vi "termalImage 01.vi"() -> ()   [LabVIEW 2018]
doc: "This example performs writes and reads on a serial port, as directed by the user. You can press the Write and Read buttons, and change the Read Count, while the example is running.\n\nThe parameters set for the serial port must match the parameters of the connected instrument or device. In this example, the Read Count parameter specifies the number of bytes that the serial port reads. If there were more bytes at the port than the specified number, those bytes would not be read. If there were less bytes at the port than the specified number, you would receive a timeout error.\n\nThis example expands upon the flow control options for XON and XOFF, allowing the user to choose those control characters. Also, the user can enable or disable a termination character. Some devices require a termination character in order to identify the end of command strings. Some devices send a termination character to signify the end of data to be read. This example shows how you can end the Read operation once a termination character is detected in the buffer and/or append a termination character at the end of the Write data."
uses:
  <vilib>/userdefined/High Color/IMAQdx.ctl
  <vilib>/Instr/_visa.llb/VISA Configure Serial Port (Instr).vi
  <vilib>/vision/driver/NI_Vision_Acquisition_Software.lvlib
  <vilib>/vision/NI_Vision_Development_Module.lvlib
panel:
  out "Cam  2":T1(plugin-control)
  in  "Camera":T2="cam1"
  in  "stop":bool
  in  "stop 2":bool
  in  "폭":dbl=10.0
  in  "중심":dbl=35.0
  out "Temperature":dbl[][](graph)
  in  "Stop":bool
  in  "VISA resource name":refnum<visa-resource-name>="COM6"
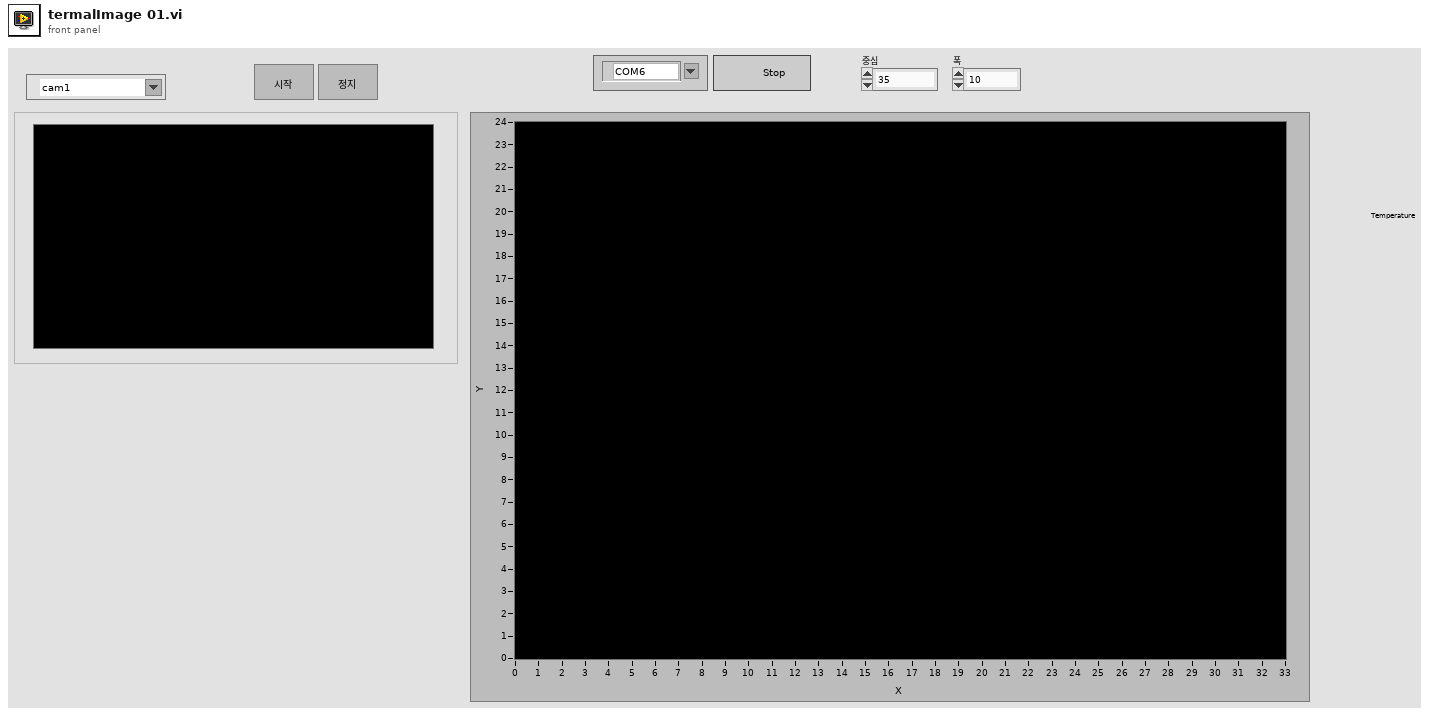
[diagram p1: front panel]
types:
  T1 = typedef "IMAQ Image.ctl" = refnum<image>
  T2 = typedef "IMAQdx.ctl" = refnum<k21>
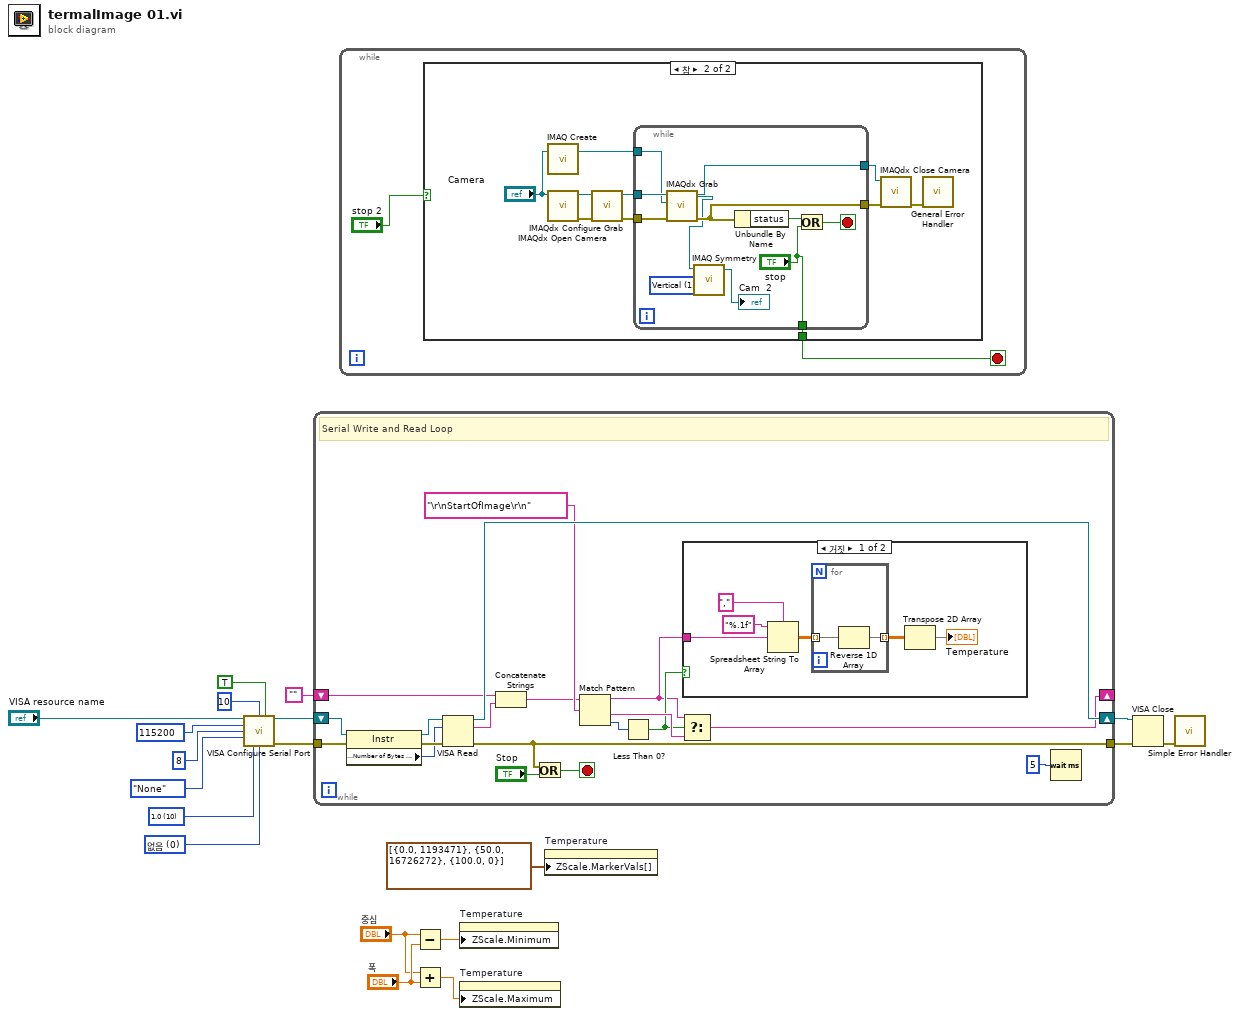
[diagram p0: block diagram]
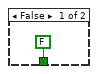
[diagram p2: hidden frame]
diagram:
  w6 = u16 0 items=["없음", "XON/XOFF", "RTS/CTS", "XON/XOFF & RTS/CTS", "DTR/DSR", "XON/XOFF & DTR/DSR"] ("flow control (0:none)")
  w7 = u16 10 items=["1.0"=10, "1.5"=15, "2.0"=20] ("stop bits (10: 1 bit)")
  n1 = call-poly "VISA Configure Serial Port"("VISA resource name"="VISA resource name", "termination char\n(0xA = '\\n' = LF)"=u8 10 ("Termination Character"), "Enable Termination\nChar (T)"=TRUE ("End Read on Termination Character?"), "baud rate (9600)"=u32 115200, "data bits (8)"=u16 8, "parity (0:none)"=enum16{"None", "Odd", "Even", "Mark", "Space"}."None", "stop bits (10: 1 bit)"=w7, "flow control (0:none)"=w6) -> ("VISA resource name out"=w13:refnum<visa-resource-name>, "error out"=w12:errorcluster)  [unwired: 2 in, 4 out]
  n2 = while {
    shift-right: [w33] -> w15
    shift-left: w13 -> [w35]
    tunnel: w12 -> [w31]
    tunnel: [w27] -> w16
    shift-right: [w20] -> _
    shift-left: "" -> [w29]
    stop <- w37 stop-if-true
    # "Serial Write and Read Loop"
    n3 = property class="Instr"(reference=w35, error in=w31) -> (reference out=w34:refnum<visa-resource-name>, error out=w32:errorcluster, "Serial Settings:Number of Bytes at Serial Port"=w30:u32)
    n4 = VISA Read(VISA resource name=w34, byte count=w30, error in (no error)=w32) -> (VISA resource name out=w33:refnum<visa-resource-name>, read buffer=w28:string, error out=w27:errorcluster)  [unwired: 1 out]
    n5 = Concatenate Strings(w29, w28) -> (w25:string)
    n6 = Or(x=w27, y="Stop") -> (x .or. y?=w37:bool)
    n7 = Match Pattern(string=w25, regular expression="\r\nStartOfImage\r\n") -> (before substring=w21:string, after substring=w23:string, offset past match=w24:i32)  [unwired: 1 in, 1 out]
    n8 = Less Than 0?(x=w24) -> (x < 0?=w22:bool)
    n9 = Select(t=w21, s=w22, f=w23) -> (s? t:f=w20:string)
    n10 = case shown="거짓" w22 {
      tunnel: w21 -> [w43 _]
      frame False {
        n11 = Spreadsheet String To Array(delimiter (Tab)=",", format string="%.1f", spreadsheet string=w43) -> (array=w41:dbl[][])  [unwired: 1 in]
        n12 = for {
          tunnel: w41 -> [w46] mode=indexing
          tunnel: [w45] -> w39 mode=indexing
          n13 = Reverse 1D Array(array=w46) -> (reversed array=w45:dbl[])
        }
        n14 = Transpose 2D Array(2D array=w39) -> (transposed array=→"Temperature":dbl[][])
      }
      frame True {
      }
    }
    n15 = Wait (ms)(milliseconds to wait=u32 5) -> ()  [unwired: 1 out]
  }
  n16 = while {
    stop <- w47 stop-if-true
    n17 = case shown="참" "stop 2" {
      tunnel: [FALSE ("stop") w50] -> w47
      frame False {
      }
      frame True {
        n18 = call "IMAQ Create"("Image Name"="Camera") -> ("New Image"=w59:T1)  [unwired: 3 in, 2 out]
        n19 = call <vilib>:"IMAQdx Open Camera.vi"("Session In"="Camera") -> ("error out"=w53:errorcluster, "Session Out"=w55:T2)  [unwired: 2 in, 7 out]
        n20 = call <vilib>:"IMAQdx Configure Grab.vi"("error in"=w53, "Session In"=w55) -> ("error out"=w51:errorcluster, "Session Out"=w52:T2)  [unwired: 1 in, 7 out]
        n21 = while {
          tunnel: [w65] -> w58
          tunnel: w51 -> [w67]
          tunnel: w52 -> [w68]
          tunnel: [w64] -> w57
          tunnel: w59 -> [w66]
          tunnel: ["stop"] -> w50
          stop <- w70 stop-if-true
          w60 = u32 1 items=["Horizontal", "Vertical", "Central", "1st Diagonal", "2nd Diagonal"] ("Type of Symmetry")
          n22 = call <vilib>:"IMAQdx Grab.vi"("error in"=w67, "Image In"=w66, "Session In"=w68) -> ("error out"=w64:errorcluster, "Image Out"=w62:T1, "Session Out"=w65:T2)  [unwired: 5 in, 1 out]
          n23 = call "IMAQ Symmetry"("Type of Symmetry"=w60, "Image Src"=w62) -> ("Image Dst Out"=→"Cam  2":T1)  [unwired: 3 in, 1 out]
          n24 = Unbundle By Name(w64) -> ("status"=w69:bool)
          n25 = Or(x=w69, y="stop") -> (x .or. y?=w70:bool)
        }
        n26 = call <vilib>:"IMAQdx Close Camera.vi"("error in"=w57, "Session In"=w58) -> ("error out"=w56:errorcluster)  [unwired: 9 out]
        n27 = call <vilib>:"General Error Handler.vi"("error in (no error)"=w56) -> ()  [unwired: 2 in, 13 out]
      }
    }
  }
  n28 = Subtract(x="중심", y="폭") -> (x-y=w5:dbl)
  n29 = Add(x="중심", y="폭") -> (x+y=w1:dbl)
  n30 = property on="Temperature" class="IntGraph (엄격한)"("ZScale.Minimum"=w5) -> ()  [unwired: 2 in, 2 out]
  n31 = property on="Temperature" class="IntGraph (엄격한)"("ZScale.Maximum"=w1) -> ()  [unwired: 2 in, 2 out]
  n32 = property on="Temperature" class="IntGraph (엄격한)"("ZScale.MarkerVals[]"=cluster{dbl, u32}[] [{0.0, 1193471}, {50.0, 16726272}, {100.0, 0}] ("Z 스케일.마커 값[]")) -> ()  [unwired: 2 in, 2 out]
  n33 = VISA Close(VISA resource name=w15, error in (no error)=w16) -> (error out=w17:errorcluster)
  n34 = call <vilib>:"Simple Error Handler.vi"("error in (no error)"=w17) -> ()  [unwired: 1 in, 8 out]
